vi "DHE_read_tp.vi"(0 "fd":i32, 1 "board":string, 2 "memory":string, 3 "address":i32, 11 "error in (no error)":errorcluster, 12 "name":string, 13 "type":string) -> (4 "fd out":i32, 8 "return value":string, 10 "busy":bool, 15 "error out":errorcluster)   [LabVIEW 2016]
doc: "This VI closes the I/O interface with the instrument."
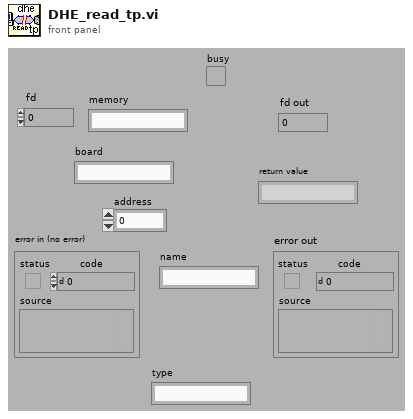
[diagram p1: front panel]
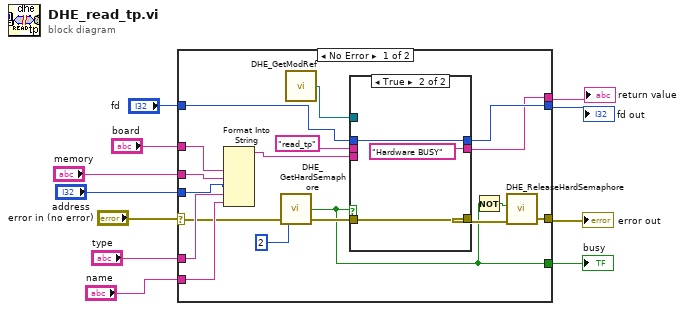
[diagram p0: block diagram]
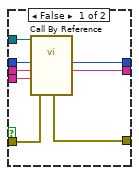
[diagram p2: hidden frame]
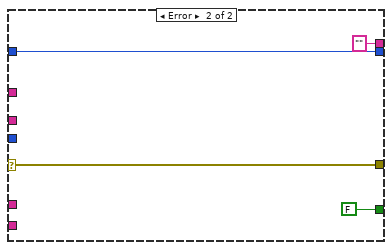
[diagram p3: hidden frame]
diagram:
  n1 = case shown="No Error" "error in (no error)" {
    selector: "error in (no error)" -> [w18 w43]
    tunnel: "fd" -> [w27 w44]
    tunnel: [w21 "" ("str result")] -> w10
    tunnel: [w15 w43] -> w9
    tunnel: [w26 w44] -> w8
    tunnel: "board" -> [w25 _]
    tunnel: "memory" -> [w24 _]
    tunnel: "address" -> [w23 _]
    tunnel: "type" -> [w20 _]
    tunnel: "name" -> [w19 _]
    tunnel: [w13 FALSE ("timed out")] -> w1
    frame No Error {
      n2 = Format Into String(w25, w24, w23, w20, w19) -> (resulting string=w22:string)  [unwired: 3 in, 1 out]
      n3 = call "DHE_GetHardSemaphore.vi"("timeout"=2, "error in (no error)"=w18) -> ("timed out"=w13:bool, "error out"=w17:errorcluster)  [unwired: 6 out]
      n4 = call "DHE_GetModRef.vi"() -> ("DHE_ModRef"=w29:refnum<vi>)  [unwired: 9 out]
      n5 = case shown="True" w13 {
        tunnel: w29 -> [w37 _]
        tunnel: "read_tp" ("function") -> [w36 _]
        tunnel: w27 -> [w35 w40]
        tunnel: [w34 w40] -> w26
        tunnel: w22 -> [w33 _]
        tunnel: [w32 "Hardware BUSY" ("str result")] -> w21
        tunnel: w17 -> [w31 w39]
        tunnel: [w30 w39] -> w16
        frame False {
          n6 = call-by-ref "?"(reference=w37, "error in (no error)"=w31, "arguments"=w33, "function"=w36, "fd in"=w35) -> ("error out"=w30:errorcluster, "str result"=w32:string, "fd out"=w34:i32)  [unwired: 5 in, 3 out]
        }
        frame True {
        }
      }
      n7 = Not(x=w13) -> (.not. x?=w12:bool)
      n8 = call "DHE_ReleaseHardSemaphore.vi"("error in (no error)"=w16, "release?"=w12) -> ("error out"=w15:errorcluster)  [unwired: 9 out]
    }
    frame Error {
    }
  }
  "error out" <- w9
  "return value" <- w10
  "fd out" <- w8
  "busy" <- w1
